vi "Kesight(7_.5) Multimeter.vi"(0 "VISA Refnum in":refnum<visa-resource-name>="USB0::0x2A8D::0x0201::MY54701494::INSTR", 1 "Operation":enum16{"Configure", "Measure"}(ring)=enum."Measure", 2 "Measurement Function (10: Voltage DC)":i32(ring)=10 items=["Continuity", "Current AC", "Current DC", "Diode", "Frequency", "Resistance 4-wire", "Period", "Resistance 2-wire", "Temperature", "Voltage AC", "Voltage DC", "Voltage DC Ratio", "Capacitance"], 5 "error in (no error)":errorcluster, 6 "ID Query (True)":bool, 7 "Sample Count (1)":i32=20, 8 "Reset (True)":bool, 10 "Auto Range (T: Enable)":bool, 11 "Timeout (10000 ms)":i32=10000, 12 "Current Integration Time (10: 10)":dbl=10.0, 13 "Manual Range (1)":dbl=1e-05) -> (14 "VISA resource name out":refnum<visa-resource-name>, 15 "Mean":dbl, 16 "Measurements":dbl[](array[numeric]), 19 "error out":errorcluster)   [LabVIEW 2019]
uses:
  <userlib>/_TI-LA/Instr Drivers/Multimeter/Agilent 3446X Series/Public/Data/Read (Multiple Points).vi
  <userlib>/_TI-LA/Instr Drivers/Multimeter/Agilent 3446X Series/Agilent 3446X Series.lvlib
panel:
  in  "Tab Control":enum32{"Config", "Measure"}(tab)
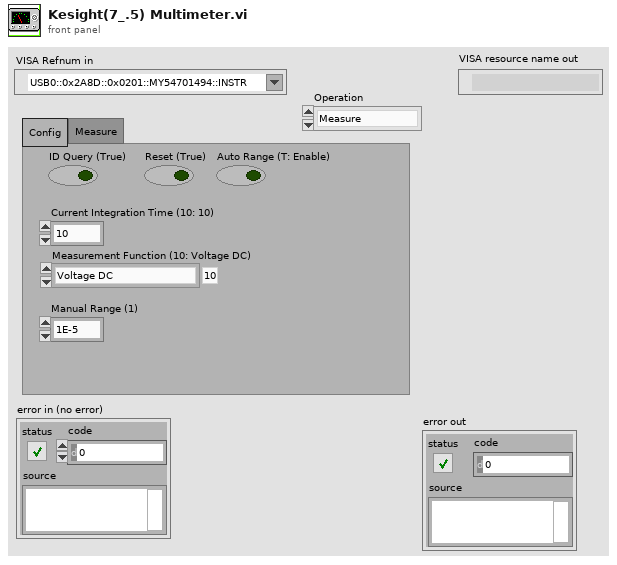
[diagram p1: front panel]
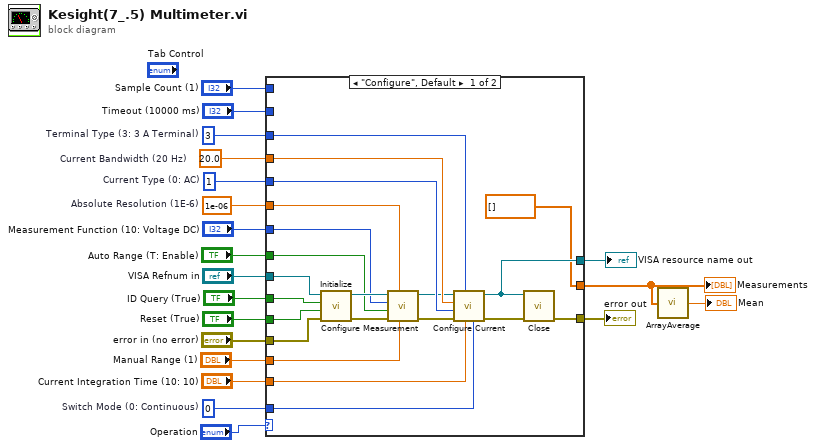
[diagram p0: block diagram]
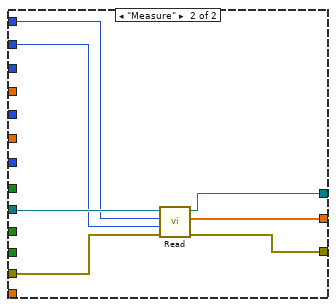
[diagram p2: hidden frame]
diagram:
  w18 = 0  # Switch Mode (0: Continuous)
  w13 = 1e-06  # Absolute Resolution (1E-6)
  w16 = 1  # Current Type (0: AC)
  w15 = 20.0  # Current Bandwidth (20 Hz)
  w14 = 3  # Terminal Type (3: 3 A Terminal)
  n1 = case shown="\"Configure\", Default" "Operation" {
    tunnel: "error in (no error)" -> [w41 w45]
    tunnel: "VISA Refnum in" -> [w40 w46]
    tunnel: w18 -> [w37 _]
    tunnel: "Current Integration Time (10: 10)" -> [w36 _]
    tunnel: w16 -> [w35 _]
    tunnel: w15 -> [w34 _]
    tunnel: w14 -> [w33 _]
    tunnel: w13 -> [w30 _]
    tunnel: "Auto Range (T: Enable)" -> [w29 _]
    tunnel: "Manual Range (1)" -> [w28 _]
    tunnel: "Sample Count (1)" -> [_ w44]
    tunnel: "Timeout (10000 ms)" -> [_ w43]
    tunnel: "ID Query (True)" -> [w27 _]
    tunnel: "Reset (True)" -> [w26 _]
    tunnel: [w24 w48] -> w6
    tunnel: [w23 w47] -> w5
    tunnel: [dbl[] [] ("Measurements") w42] -> w4
    tunnel: "Measurement Function (10: Voltage DC)" -> [w21 _]
    frame "Configure", Default {
      n2 = call <userlib>:"Initialize.vi"("error in (no error)"=w41, "Reset (True)"=w26, "ID Query (True)"=w27, "VISA resource name"=w40) -> ("error out"=w38:errorcluster, "VISA resource name out"=w39:refnum<visa-resource-name>)  [unwired: 6 in]
      n3 = call <userlib>:"Configure Measurement.vi"("Manual Range (1)"=w28, "Absolute Resolution (1E-6)"=w30, "error in (no error)"=w38, "Auto Range (T: Enable)"=w29, "Measurement Function (10: Voltage DC)"=w21, "VISA resource name"=w39) -> ("error out"=w32:errorcluster, "VISA resource name out"=w31:refnum<visa-resource-name>)  [unwired: 4 in]
      n4 = call <userlib>:"Configure Current.vi"("Switch Mode (0: Continuous)"=w37, "Current Integration Time (10: 10)"=w36, "Terminal Type (3: 3 A Terminal)"=w33, "error in (no error)"=w32, "Current Type (0: AC)"=w35, "Current Bandwidth (20 Hz)"=w34, "VISA resource name"=w31) -> ("error out"=w25:errorcluster, "VISA resource name out"=w24:refnum<visa-resource-name>)  [unwired: 3 in]
      n5 = call <userlib>:"Close.vi"("error in (no error)"=w25, "VISA resource name"=w24) -> ("error out"=w23:errorcluster)  [unwired: 9 in]
    }
    frame "Measure" {
      n6 = call-poly <userlib>:"Read.vi"("error in (no error)"=w45, "Timeout (10000 ms)"=w43, "Sample Count (1)"=w44, "VISA resource name"=w46) -> ("error out"=w47:errorcluster, "Measurements"=w42:dbl[], "VISA resource name out"=w48:refnum<visa-resource-name>)  [unwired: 5 in]
    }
  }
  "Measurements" <- w4
  "VISA resource name out" <- w6
  "error out" <- w5
  n7 = call "ArrayAverage.vi"("InputArray"=w4) -> ("AvgOut"=→"Mean":dbl)  [unwired: 4 in]
